vi "Windows Main-forextreme.vi"() -> ()   [LabVIEW 2016]
uses:
  <resource>/objmgr/ni.dex.rc
panel:
  out "Array 10":i32[][](array[numeric])
  in  "停止应用程序 11":bool
  in  "停止应用程序 10":bool
  out "Array 9":i32[][](array[numeric])
  in  "停止应用程序 9":bool
  out "Gaussian2-4":T1(plugin-control)
  out "Array 8":i32[][](array[numeric])
  in  "停止应用程序 8":bool
  out "Gaussian2-3":T1(plugin-control)
  out "Array 7":i32[][](array[numeric])
  in  "停止应用程序 7":bool
  out "Gaussian2-2":T1(plugin-control)
  out "Array 6":i32[][](array[numeric])
  in  "停止应用程序 6":bool
  out "Gaussian2-1":T1(plugin-control)
  out "Array 5":i32[][](array[numeric])
  in  "停止应用程序 5":bool
  out "Gaussian1-4":T1(plugin-control)
  out "Array 4":i32[][](array[numeric])
  in  "停止应用程序 4":bool
  out "Gaussian1-3":T1(plugin-control)
  out "Array 3":i32[][](array[numeric])
  in  "停止应用程序 3":bool
  out "Gaussian1-2":T1(plugin-control)
  out "Array 2":i32[][](array[numeric])
  out "error out 2":errorcluster
  in  "停止应用程序 2":bool
  out "OriImage":T1(plugin-control)
  out "Array":i32[][](array[numeric])
  out "Numeric":i32
  in  "终端IP地址":string
  out "error out":errorcluster
  in  "停止应用程序":bool
  out "Gaussian1-1":T1(plugin-control)
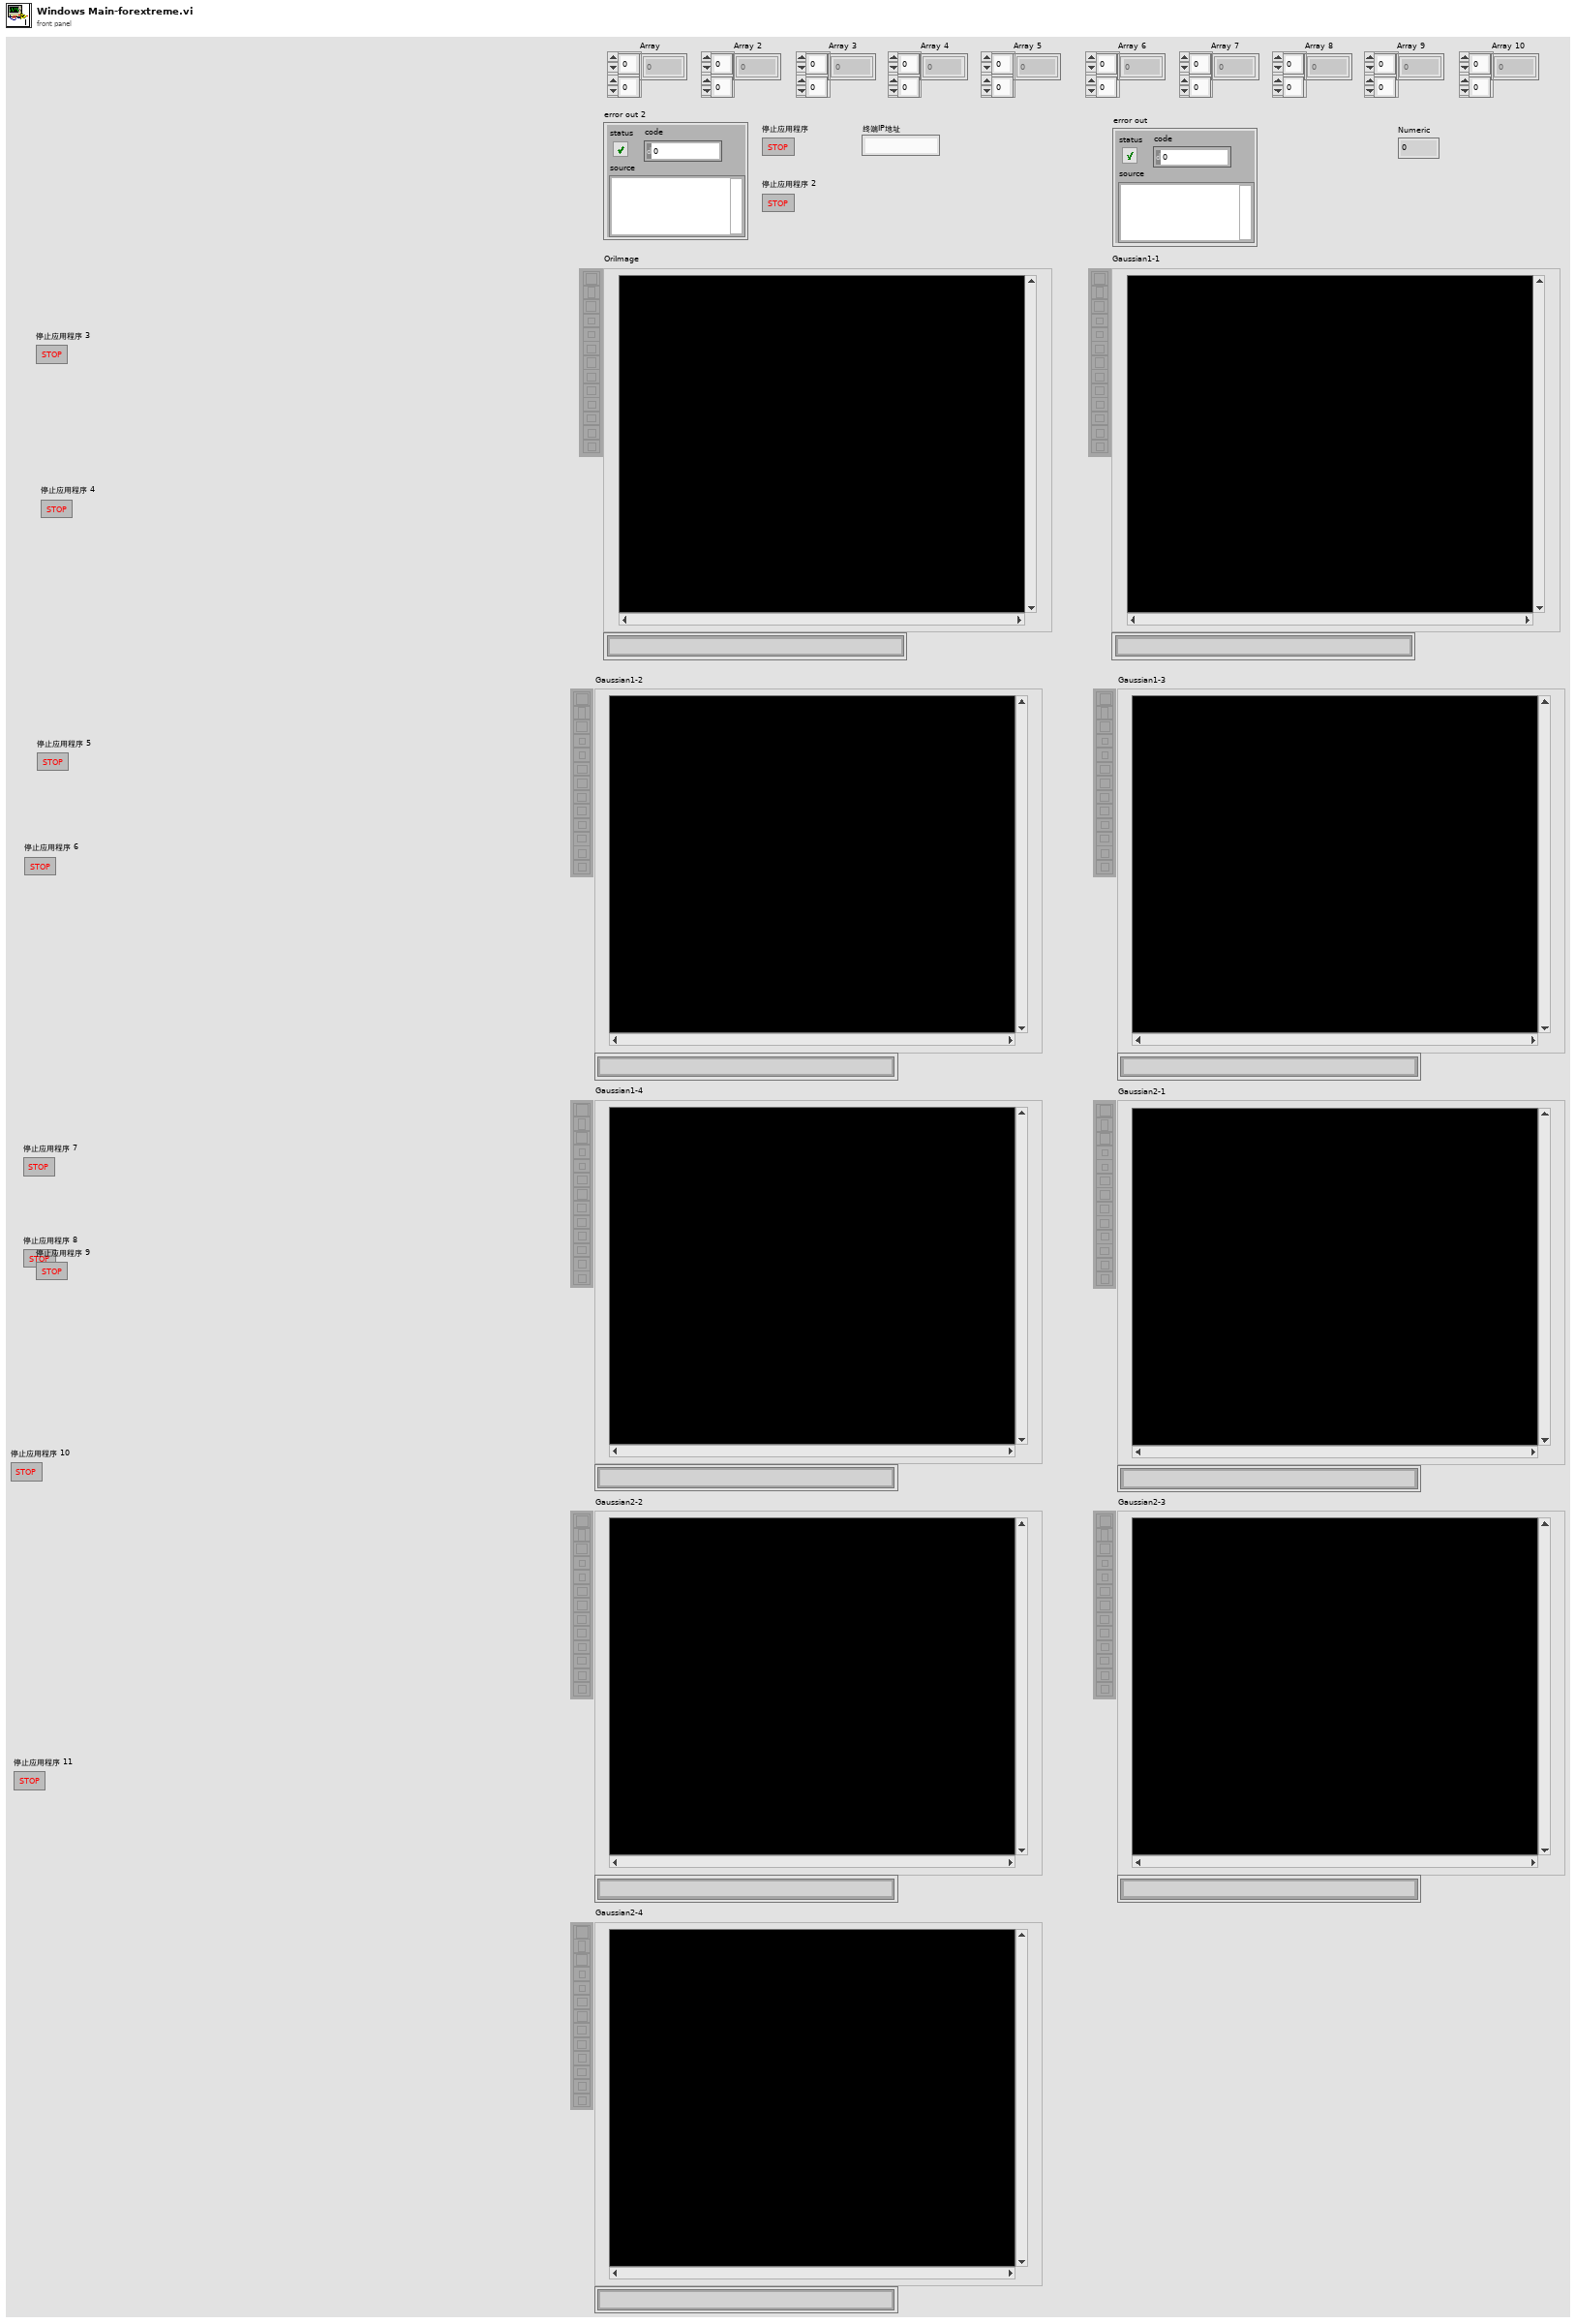
[diagram p1: front panel]
types:
  T1 = typedef "IMAQ Image.ctl" = refnum<image>
  T2 = typedef "Image Type" = u32
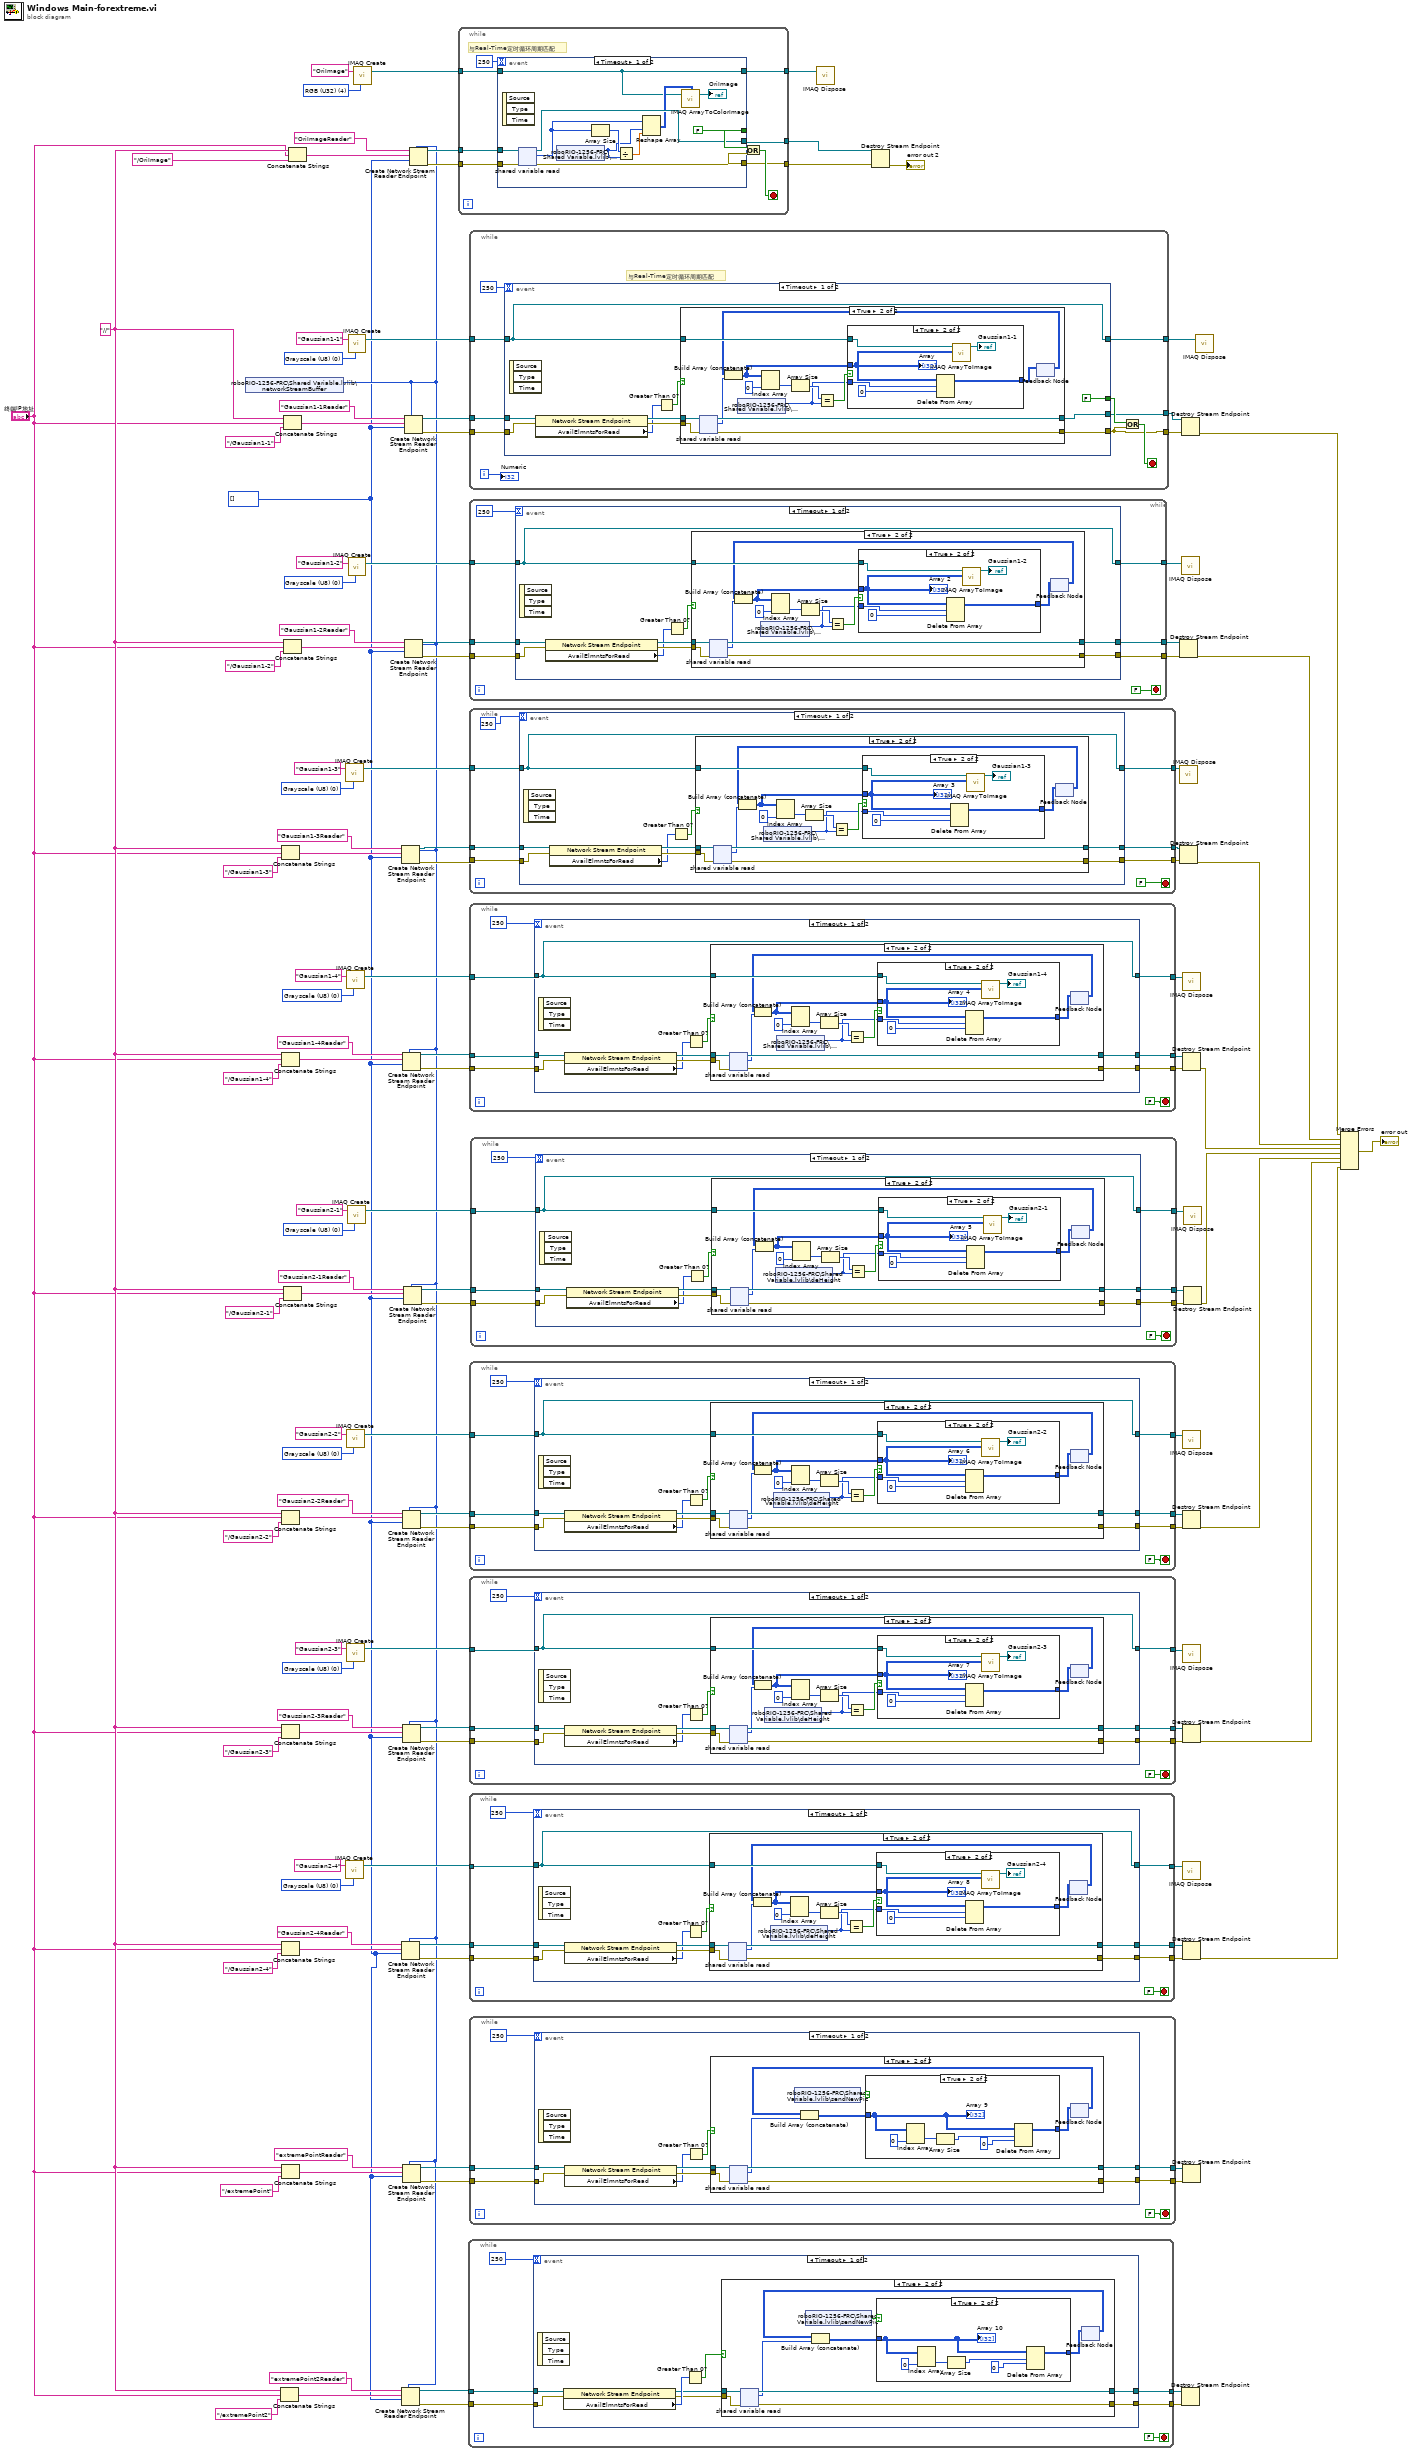
[diagram p0: block diagram]
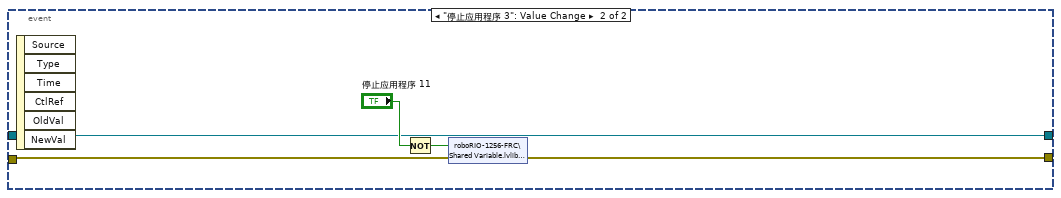
[diagram p4: hidden frame]
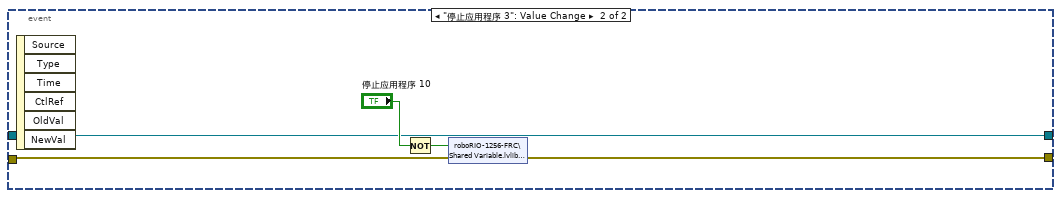
[diagram p7: hidden frame]
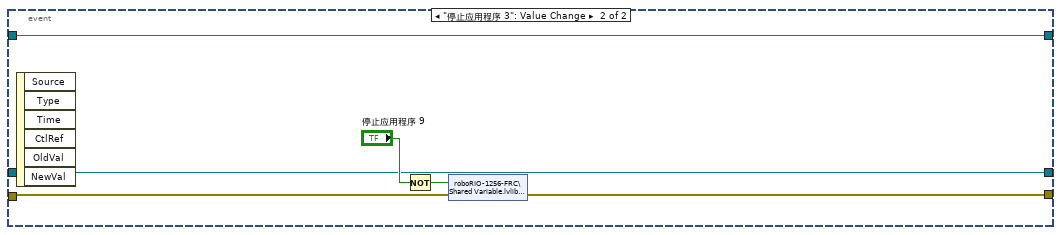
[diagram p10: hidden frame]
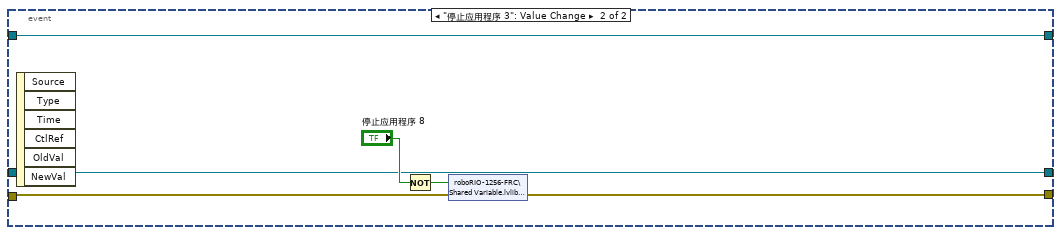
[diagram p13: hidden frame]
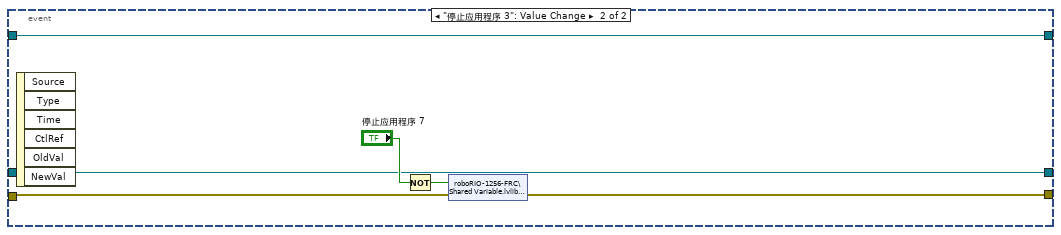
[diagram p16: hidden frame]
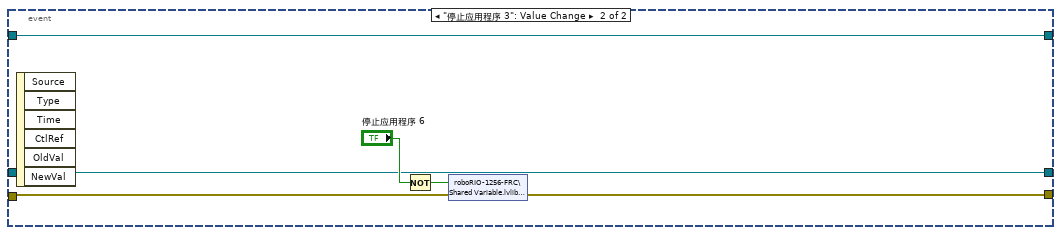
[diagram p19: hidden frame]
diagram:
  w32 = T2 0 items=["Grayscale (U8)", "Grayscale (I16)", "Grayscale (SGL)", "Complex (CSG)", "RGB (U32)", "HSL (U32)", "RGB (U64)", "Grayscale (U16)"] ("Image Type")
  w33 = T2 0 items=["Grayscale (U8)", "Grayscale (I16)", "Grayscale (SGL)", "Complex (CSG)", "RGB (U32)", "HSL (U32)", "RGB (U64)", "Grayscale (U16)"] ("Image Type")
  w54 = T2 0 items=["Grayscale (U8)", "Grayscale (I16)", "Grayscale (SGL)", "Complex (CSG)", "RGB (U32)", "HSL (U32)", "RGB (U64)", "Grayscale (U16)"] ("Image Type")
  w56 = T2 0 items=["Grayscale (U8)", "Grayscale (I16)", "Grayscale (SGL)", "Complex (CSG)", "RGB (U32)", "HSL (U32)", "RGB (U64)", "Grayscale (U16)"] ("Image Type")
  w90 = T2 0 items=["Grayscale (U8)", "Grayscale (I16)", "Grayscale (SGL)", "Complex (CSG)", "RGB (U32)", "HSL (U32)", "RGB (U64)", "Grayscale (U16)"] ("Image Type")
  w95 = T2 0 items=["Grayscale (U8)", "Grayscale (I16)", "Grayscale (SGL)", "Complex (CSG)", "RGB (U32)", "HSL (U32)", "RGB (U64)", "Grayscale (U16)"] ("Image Type")
  w96 = T2 0 items=["Grayscale (U8)", "Grayscale (I16)", "Grayscale (SGL)", "Complex (CSG)", "RGB (U32)", "HSL (U32)", "RGB (U64)", "Grayscale (U16)"] ("Image Type")
  w108 = T2 4 items=["Grayscale (U8)", "Grayscale (I16)", "Grayscale (SGL)", "Complex (CSG)", "RGB (U32)", "HSL (U32)", "RGB (U64)", "Grayscale (U16)"] ("Image Type")
  w101 = T2 0 items=["Grayscale (U8)", "Grayscale (I16)", "Grayscale (SGL)", "Complex (CSG)", "RGB (U32)", "HSL (U32)", "RGB (U64)", "Grayscale (U16)"] ("Image Type")
  w3 = i32[] []
  w2 = "//" ("string")
  n1 = shared-variable "roboRIO-1256-FRC\\Shared Variable.lvlib\\networkStreamBuffer"() -> (w4:i8)  [unwired: 1 in, 1 out]
  n2 = Concatenate Strings(w2, "终端IP地址", "/extremePoint2" ("string")) -> (w9:string)
  n3 = Concatenate Strings(w2, "终端IP地址", "/Gaussian1-3" ("string")) -> (w99:string)
  n4 = Concatenate Strings(w2, "终端IP地址", "/Gaussian2-4" ("string")) -> (w29:string)
  n5 = Concatenate Strings(w2, "终端IP地址", "/Gaussian1-4" ("string")) -> (w87:string)
  n6 = Concatenate Strings(w2, "终端IP地址", "/Gaussian2-2" ("string")) -> (w51:string)
  n7 = Concatenate Strings(w2, "终端IP地址", "/Gaussian2-3" ("string")) -> (w36:string)
  n8 = Concatenate Strings(w2, "终端IP地址", "/extremePoint" ("string")) -> (w14:string)
  n9 = Concatenate Strings(w2, "终端IP地址", "/Gaussian2-1" ("string")) -> (w59:string)
  n10 = Concatenate Strings(w2, "终端IP地址", "/Gaussian1-1" ("string")) -> (w124:string)
  n11 = Concatenate Strings(w2, "终端IP地址", "/Gaussian1-2" ("string")) -> (w103:string)
  n12 = Concatenate Strings(w2, "终端IP地址", "/OriImage" ("string")) -> (w114:string)
  n13 = call "IMAQ Create"("Image Name"="Gaussian1-3", "Image Type"=w95) -> ("New Image"=w78:T1)  [unwired: 3 in, 1 out]
  n14 = call "IMAQ Create"("Image Name"="Gaussian2-4", "Image Type"=w32) -> ("New Image"=w27:T1)  [unwired: 3 in, 1 out]
  n15 = call "IMAQ Create"("Image Name"="Gaussian1-4", "Image Type"=w90) -> ("New Image"=w84:T1)  [unwired: 3 in, 1 out]
  n16 = call "IMAQ Create"("Image Name"="Gaussian2-2", "Image Type"=w54) -> ("New Image"=w49:T1)  [unwired: 3 in, 1 out]
  n17 = call "IMAQ Create"("Image Name"="Gaussian2-3", "Image Type"=w33) -> ("New Image"=w38:T1)  [unwired: 3 in, 1 out]
  n18 = call "IMAQ Create"("Image Name"="Gaussian2-1", "Image Type"=w56) -> ("New Image"=w61:T1)  [unwired: 3 in, 1 out]
  n19 = call "IMAQ Create"("Image Name"="Gaussian1-1", "Image Type"=w101) -> ("New Image"=w120:T1)  [unwired: 3 in, 1 out]
  n20 = call "IMAQ Create"("Image Name"="Gaussian1-2", "Image Type"=w96) -> ("New Image"=w70:T1)  [unwired: 3 in, 1 out]
  n21 = call "IMAQ Create"("Image Name"="OriImage", "Image Type"=w108) -> ("New Image"=w107:T1)  [unwired: 3 in, 1 out]
  n22 = Create Network Stream Reader Endpoint(7:w4, 9:w3, 10:w9, 11:"extremePoint2Reader" ("reader name")) -> (0:w7:errorcluster, 3:w8:refnum<k21>)  [unwired: 3 in]
  n23 = Create Network Stream Reader Endpoint(7:w4, 9:w3, 10:w99, 11:"Gaussian1-3Reader" ("reader name")) -> (0:w76:errorcluster, 3:w77:refnum<k21>)  [unwired: 3 in]
  n24 = Create Network Stream Reader Endpoint(7:w4, 9:w3, 10:w29, 11:"Gaussian2-4Reader" ("reader name")) -> (0:w25:errorcluster, 3:w26:refnum<k21>)  [unwired: 3 in]
  n25 = Create Network Stream Reader Endpoint(7:w4, 9:w3, 10:w87, 11:"Gaussian1-4Reader" ("reader name")) -> (0:w82:errorcluster, 3:w83:refnum<k21>)  [unwired: 3 in]
  n26 = Create Network Stream Reader Endpoint(7:w4, 9:w3, 10:w51, 11:"Gaussian2-2Reader" ("reader name")) -> (0:w47:errorcluster, 3:w48:refnum<k21>)  [unwired: 3 in]
  n27 = Create Network Stream Reader Endpoint(7:w4, 9:w3, 10:w36, 11:"Gaussian2-3Reader" ("reader name")) -> (0:w40:errorcluster, 3:w39:refnum<k21>)  [unwired: 3 in]
  n28 = Create Network Stream Reader Endpoint(7:w4, 9:w3, 10:w14, 11:"extremePointReader" ("reader name")) -> (0:w16:errorcluster, 3:w15:refnum<k21>)  [unwired: 3 in]
  n29 = Create Network Stream Reader Endpoint(7:w4, 9:w3, 10:w59, 11:"Gaussian2-1Reader" ("reader name")) -> (0:w63:errorcluster, 3:w62:refnum<k21>)  [unwired: 3 in]
  n30 = Create Network Stream Reader Endpoint(7:w4, 9:w3, 10:w124, 11:"Gaussian1-1Reader" ("reader name")) -> (0:w127:errorcluster, 3:w118:refnum<k21>)  [unwired: 3 in]
  n31 = Create Network Stream Reader Endpoint(7:w4, 9:w3, 10:w103, 11:"Gaussian1-2Reader" ("reader name")) -> (0:w71:errorcluster, 3:w72:refnum<k21>)  [unwired: 3 in]
  n32 = Create Network Stream Reader Endpoint(7:w4, 9:w3, 10:w114, 11:"OriImageReader" ("reader name")) -> (0:w117:errorcluster, 3:w112:refnum<k21>)  [unwired: 3 in]
  n33 = while {
    tunnel: w112 -> [w131]
    tunnel: [w130] -> w111
    tunnel: w107 -> [w129]
    tunnel: [w128] -> w106
    tunnel: w117 -> [w133]
    tunnel: [w132] -> w113
    stop <- w134 stop-if-true
    # "与Real-Time定时循环周期匹配"
    n34 = event shown="[0] Timeout" {
      selector: _ -> [_ _]
      dyn-events: _ -> [_ _]
      timeout: 250 -> [_ _]
      tunnel: [FALSE ("停止应用程序") "停止应用程序 2"] -> w135
      tunnel: w133 -> [w148 w152]
      tunnel: [w147 w151] -> w132
      tunnel: w131 -> [w146 w149]
      tunnel: [w145 w149] -> w130
      tunnel: w129 -> [w138 w150]
      tunnel: [w138 w150] -> w128
      event Timeout {
        n35 = event-data() -> ()  [unwired: 1 in, 3 out]
        n36 = shared-variable-read(w146, w148) -> (w145:refnum<k21>, w147:errorcluster, w141:i32[])  [unwired: 1 in, 1 out]
        n37 = shared-variable "roboRIO-1256-FRC\\Shared Variable.lvlib\\Height"() -> (w137:u16)  [unwired: 1 in, 1 out]
        n38 = Array Size(array=w141) -> (size(s)=w143:i32)
        n39 = Divide(x=w143, y=w137) -> (x/y=w142:dbl)
        n40 = Reshape Array(w141, w137, w142) -> (w140:i32[][])
        n41 = call "IMAQ ArrayToColorImage"("Image Pixels (U32)"=w140, "Image"=w138) -> ("Image Out"=→"OriImage":T1)  [unwired: 3 in, 1 out]
      }
      event "停止应用程序 2": Value Change {
        n42 = event-data() -> ()  [unwired: 1 in, 6 out]
        n43 = Not(x="停止应用程序 2") -> (.not. x?=w153:bool)
        n44 = shared-variable "roboRIO-1256-FRC\\Shared Variable.lvlib\\Active"(w153, error in=w152) -> (error out=w151:errorcluster)
      }
    }
    n45 = Or(x=w135, y=w132) -> (x .or. y?=w134:bool)
  }
  n46 = while {
    tunnel: w8 -> [w160]
    tunnel: [w157] -> w5
    tunnel: w7 -> [w159]
    tunnel: [w158] -> w6
    stop <- FALSE stop-if-true
    n47 = event shown="[0] Timeout" {
      selector: _ -> [_ _]
      dyn-events: _ -> [_ _]
      timeout: 250 -> [_ _]
      tunnel: w159 -> [w168 w189]
      tunnel: [w161 w188] -> w158
      tunnel: w160 -> [w167 w187]
      tunnel: [w162 w187] -> w157
      event Timeout {
        n48 = event-data() -> ()  [unwired: 1 in, 3 out]
        n49 = property class="Network Stream Endpoint"(reference=w167, error in=w168) -> (reference out=w165:refnum<k21>, error out=w164:errorcluster, "AvailElmntsForRead"=w166:i32)
        n50 = Greater Than 0?(x=w166) -> (x > 0?=w163:bool)
        n51 = case shown="True" w163 {
          tunnel: [w169 w179] -> w161
          tunnel: [w170 w178] -> w162
          tunnel: w164 -> [w169 w177]
          tunnel: w165 -> [w170 w176]
          frame False {
          }
          frame True {
            n52 = shared-variable-read(w176, w177) -> (w178:refnum<k21>, w179:errorcluster, w175:i32[])  [unwired: 1 in, 1 out]
            n53 = shared-variable "roboRIO-1256-FRC\\Shared Variable.lvlib\\sendNewPic"() -> (w171:bool)  [unwired: 1 in, 1 out]
            n54 = feedback #1() -> (w173:i32[][])  [unwired: 1 in]
            n55 = Build Array (concatenate)(w173, w175) -> (w172:i32[][])
            n56 = case shown="True" w171 {
              tunnel: w172 -> [w180 w181]
              tunnel: [w180 w185] -> w174
              frame False {
              }
              frame True {
                n57 = Index Array(array=w181, index (col)=0 ("disabled index (col)")) -> (element=w184:i32[])  [unwired: 1 in]
                n58 = Array Size(array=w184) -> (size(s)=w182:i32)
                n59 = Delete From Array(array=w181, length=w182, index (row)=0) -> (array with subset deleted=w185:i32[][])  [unwired: 1 in, 1 out]
                "Array 10" <- w181
              }
            }
            n60 = feedback-in #1(w174) -> ()
          }
        }
      }
      event "停止应用程序 3": Value Change {
        n61 = event-data() -> ()  [unwired: 1 in, 6 out]
        n62 = Not(x="停止应用程序 11") -> (.not. x?=w190:bool)
        n63 = shared-variable "roboRIO-1256-FRC\\Shared Variable.lvlib\\Active"(w190, error in=w189) -> (error out=w188:errorcluster)
      }
    }
  }
  n64 = while {
    tunnel: w27 -> [w199]
    tunnel: [w194] -> w22
    tunnel: w26 -> [w198]
    tunnel: [w195] -> w23
    tunnel: w25 -> [w197]
    tunnel: [w196] -> w24
    stop <- FALSE stop-if-true
    n65 = event shown="[0] Timeout" {
      selector: _ -> [_ _]
      dyn-events: _ -> [_ _]
      timeout: 250 -> [_ _]
      tunnel: w197 -> [w205 w235]
      tunnel: [w208 w234] -> w196
      tunnel: w198 -> [w204 w232]
      tunnel: [w207 w232] -> w195
      tunnel: w199 -> [w206 w233]
      tunnel: [w206 w233] -> w194
      event Timeout {
        n66 = event-data() -> ()  [unwired: 1 in, 3 out]
        n67 = property class="Network Stream Endpoint"(reference=w204, error in=w205) -> (reference out=w202:refnum<k21>, error out=w203:errorcluster, "AvailElmntsForRead"=w201:i32)
        n68 = Greater Than 0?(x=w201) -> (x > 0?=w200:bool)
        n69 = case shown="True" w200 {
          tunnel: [w209 w224] -> w208
          tunnel: [w210 w223] -> w207
          tunnel: w206 -> [_ w216]
          tunnel: w203 -> [w209 w218]
          tunnel: w202 -> [w210 w217]
          frame False {
          }
          frame True {
            n70 = shared-variable-read(w217, w218) -> (w223:refnum<k21>, w224:errorcluster, w214:i32[])  [unwired: 1 in, 1 out]
            n71 = shared-variable "roboRIO-1256-FRC\\Shared Variable.lvlib\\deHeight"() -> (w211:u16)  [unwired: 1 in, 1 out]
            n72 = feedback #2() -> (w212:i32[][])  [unwired: 1 in]
            n73 = Build Array (concatenate)(w212, w214) -> (w215:i32[][])
            n74 = Index Array(array=w215, index (col)=0 ("disabled index (col)")) -> (element=w221:i32[])  [unwired: 1 in]
            n75 = Array Size(array=w221) -> (size(s)=w220:i32)
            n76 = Equal?(x=w220, y=w211) -> (x = y?=w219:bool)
            n77 = case shown="True" w219 {
              tunnel: w215 -> [w225 w226]
              tunnel: [w225 w227] -> w213
              tunnel: w211 -> [_ w231]
              tunnel: w216 -> [_ w228]
              frame False {
              }
              frame True {
                n78 = Delete From Array(array=w226, length=w231, index (row)=0) -> (array with subset deleted=w227:i32[][])  [unwired: 1 in, 1 out]
                n79 = call "IMAQ ArrayToImage"("Image Pixels (U8)"=w226, "Image"=w228) -> ("Image Out"=→"Gaussian2-4":T1)  [unwired: 8 in, 1 out]
                "Array 8" <- w226
              }
            }
            n80 = feedback-in #2(w213) -> ()
          }
        }
      }
      event "停止应用程序 3": Value Change {
        n81 = event-data() -> ()  [unwired: 1 in, 6 out]
        n82 = Not(x="停止应用程序 9") -> (.not. x?=w236:bool)
        n83 = shared-variable "roboRIO-1256-FRC\\Shared Variable.lvlib\\Active"(w236, error in=w235) -> (error out=w234:errorcluster)
      }
    }
  }
  n84 = while {
    tunnel: w118 -> [w242]
    tunnel: [w241] -> w122
    tunnel: w120 -> [w240]
    tunnel: [w239] -> w119
    tunnel: w127 -> [w244]
    tunnel: [w243] -> w123
    i -> [w238]
    stop <- w245 stop-if-true
    # "与Real-Time定时循环周期匹配"
    n85 = event shown="[0] Timeout" {
      selector: _ -> [_ _]
      dyn-events: _ -> [_ _]
      timeout: 250 -> [_ _]
      tunnel: [FALSE ("停止应用程序") "停止应用程序"] -> w246
      tunnel: w244 -> [w253 w284]
      tunnel: [w257 w283] -> w243
      tunnel: w242 -> [w252 w281]
      tunnel: [w256 w281] -> w241
      tunnel: w240 -> [w254 w282]
      tunnel: [w254 w282] -> w239
      event Timeout {
        n86 = event-data() -> ()  [unwired: 1 in, 3 out]
        n87 = property class="Network Stream Endpoint"(reference=w252, error in=w253) -> (reference out=w250:refnum<k21>, error out=w251:errorcluster, "AvailElmntsForRead"=w249:i32)
        n88 = Greater Than 0?(x=w249) -> (x > 0?=w248:bool)
        n89 = case shown="True" w248 {
          tunnel: [w258 w273] -> w257
          tunnel: [w259 w272] -> w256
          tunnel: w254 -> [_ w265]
          tunnel: w251 -> [w258 w267]
          tunnel: w250 -> [w259 w266]
          frame False {
          }
          frame True {
            n90 = shared-variable-read(w266, w267) -> (w272:refnum<k21>, w273:errorcluster, w263:i32[])  [unwired: 1 in, 1 out]
            n91 = shared-variable "roboRIO-1256-FRC\\Shared Variable.lvlib\\Height"() -> (w260:u16)  [unwired: 1 in, 1 out]
            n92 = feedback #3() -> (w261:i32[][])  [unwired: 1 in]
            n93 = Build Array (concatenate)(w261, w263) -> (w264:i32[][])
            n94 = Index Array(array=w264, index (col)=0 ("disabled index (col)")) -> (element=w270:i32[])  [unwired: 1 in]
            n95 = Array Size(array=w270) -> (size(s)=w269:i32)
            n96 = Equal?(x=w269, y=w260) -> (x = y?=w268:bool)
            n97 = case shown="True" w268 {
              tunnel: w264 -> [w274 w275]
              tunnel: [w274 w276] -> w262
              tunnel: w260 -> [_ w280]
              tunnel: w265 -> [_ w277]
              frame False {
              }
              frame True {
                n98 = Delete From Array(array=w275, length=w280, index (row)=0) -> (array with subset deleted=w276:i32[][])  [unwired: 1 in, 1 out]
                n99 = call "IMAQ ArrayToImage"("Image Pixels (U8)"=w275, "Image"=w277) -> ("Image Out"=→"Gaussian1-1":T1)  [unwired: 8 in, 1 out]
                "Array" <- w275
              }
            }
            n100 = feedback-in #3(w262) -> ()
          }
        }
      }
      event "停止应用程序": Value Change {
        n101 = event-data() -> ()  [unwired: 1 in, 6 out]
        n102 = Not(x="停止应用程序") -> (.not. x?=w285:bool)
        n103 = shared-variable "roboRIO-1256-FRC\\Shared Variable.lvlib\\Active"(w285, error in=w284) -> (error out=w283:errorcluster)
      }
    }
    n104 = Or(x=w246, y=w243) -> (x .or. y?=w245:bool)
    "Numeric" <- w238
  }
  n105 = while {
    tunnel: w70 -> [w292]
    tunnel: [w291] -> w69
    tunnel: w72 -> [w294]
    tunnel: [w290] -> w68
    tunnel: w71 -> [w293]
    tunnel: [w289] -> w67
    stop <- FALSE stop-if-true
    n106 = event shown="[0] Timeout" {
      selector: _ -> [_ _]
      dyn-events: _ -> [_ _]
      timeout: 250 -> [_ _]
      tunnel: w293 -> [w300 w330]
      tunnel: [w303 w329] -> w289
      tunnel: w294 -> [w299 w327]
      tunnel: [w302 w327] -> w290
      tunnel: w292 -> [w301 w328]
      tunnel: [w301 w328] -> w291
      event Timeout {
        n107 = event-data() -> ()  [unwired: 1 in, 3 out]
        n108 = property class="Network Stream Endpoint"(reference=w299, error in=w300) -> (reference out=w297:refnum<k21>, error out=w298:errorcluster, "AvailElmntsForRead"=w296:i32)
        n109 = Greater Than 0?(x=w296) -> (x > 0?=w295:bool)
        n110 = case shown="True" w295 {
          tunnel: [w304 w319] -> w303
          tunnel: [w305 w318] -> w302
          tunnel: w301 -> [_ w311]
          tunnel: w298 -> [w304 w313]
          tunnel: w297 -> [w305 w312]
          frame False {
          }
          frame True {
            n111 = shared-variable-read(w312, w313) -> (w318:refnum<k21>, w319:errorcluster, w309:i32[])  [unwired: 1 in, 1 out]
            n112 = shared-variable "roboRIO-1256-FRC\\Shared Variable.lvlib\\Height"() -> (w306:u16)  [unwired: 1 in, 1 out]
            n113 = feedback #4() -> (w307:i32[][])  [unwired: 1 in]
            n114 = Build Array (concatenate)(w307, w309) -> (w310:i32[][])
            n115 = Index Array(array=w310, index (col)=0 ("disabled index (col)")) -> (element=w316:i32[])  [unwired: 1 in]
            n116 = Array Size(array=w316) -> (size(s)=w315:i32)
            n117 = Equal?(x=w315, y=w306) -> (x = y?=w314:bool)
            n118 = case shown="True" w314 {
              tunnel: w310 -> [w320 w321]
              tunnel: [w320 w322] -> w308
              tunnel: w306 -> [_ w326]
              tunnel: w311 -> [_ w323]
              frame False {
              }
              frame True {
                n119 = Delete From Array(array=w321, length=w326, index (row)=0) -> (array with subset deleted=w322:i32[][])  [unwired: 1 in, 1 out]
                n120 = call "IMAQ ArrayToImage"("Image Pixels (U8)"=w321, "Image"=w323) -> ("Image Out"=→"Gaussian1-2":T1)  [unwired: 8 in, 1 out]
                "Array 2" <- w321
              }
            }
            n121 = feedback-in #4(w308) -> ()
          }
        }
      }
      event "停止应用程序 3": Value Change {
        n122 = event-data() -> ()  [unwired: 1 in, 6 out]
        n123 = Not(x="停止应用程序 3") -> (.not. x?=w331:bool)
        n124 = shared-variable "roboRIO-1256-FRC\\Shared Variable.lvlib\\Active"(w331, error in=w330) -> (error out=w329:errorcluster)
      }
    }
  }
  n125 = while {
    tunnel: w78 -> [w340]
    tunnel: [w335] -> w73
    tunnel: w77 -> [w339]
    tunnel: [w337] -> w75
    tunnel: w76 -> [w338]
    tunnel: [w336] -> w74
    stop <- FALSE stop-if-true
    n126 = event shown="[0] Timeout" {
      selector: _ -> [_ _]
      dyn-events: _ -> [_ _]
      timeout: 250 -> [_ _]
      tunnel: w338 -> [w346 w376]
      tunnel: [w349 w375] -> w336
      tunnel: w339 -> [w345 w373]
      tunnel: [w348 w373] -> w337
      tunnel: w340 -> [w347 w374]
      tunnel: [w347 w374] -> w335
      event Timeout {
        n127 = event-data() -> ()  [unwired: 1 in, 3 out]
        n128 = property class="Network Stream Endpoint"(reference=w345, error in=w346) -> (reference out=w343:refnum<k21>, error out=w344:errorcluster, "AvailElmntsForRead"=w342:i32)
        n129 = Greater Than 0?(x=w342) -> (x > 0?=w341:bool)
        n130 = case shown="True" w341 {
          tunnel: [w350 w365] -> w349
          tunnel: [w351 w364] -> w348
          tunnel: w347 -> [_ w357]
          tunnel: w344 -> [w350 w359]
          tunnel: w343 -> [w351 w358]
          frame False {
          }
          frame True {
            n131 = shared-variable-read(w358, w359) -> (w364:refnum<k21>, w365:errorcluster, w355:i32[])  [unwired: 1 in, 1 out]
            n132 = shared-variable "roboRIO-1256-FRC\\Shared Variable.lvlib\\Height"() -> (w352:u16)  [unwired: 1 in, 1 out]
            n133 = feedback #5() -> (w353:i32[][])  [unwired: 1 in]
            n134 = Build Array (concatenate)(w353, w355) -> (w356:i32[][])
            n135 = Index Array(array=w356, index (col)=0 ("disabled index (col)")) -> (element=w362:i32[])  [unwired: 1 in]
            n136 = Array Size(array=w362) -> (size(s)=w361:i32)
            n137 = Equal?(x=w361, y=w352) -> (x = y?=w360:bool)
            n138 = case shown="True" w360 {
              tunnel: w356 -> [w366 w367]
              tunnel: [w366 w368] -> w354
              tunnel: w352 -> [_ w372]
              tunnel: w357 -> [_ w369]
              frame False {
              }
              frame True {
                n139 = Delete From Array(array=w367, length=w372, index (row)=0) -> (array with subset deleted=w368:i32[][])  [unwired: 1 in, 1 out]
                n140 = call "IMAQ ArrayToImage"("Image Pixels (U8)"=w367, "Image"=w369) -> ("Image Out"=→"Gaussian1-3":T1)  [unwired: 8 in, 1 out]
                "Array 3" <- w367
              }
            }
            n141 = feedback-in #5(w354) -> ()
          }
        }
      }
      event "停止应用程序 3": Value Change {
        n142 = event-data() -> ()  [unwired: 1 in, 6 out]
        n143 = Not(x="停止应用程序 4") -> (.not. x?=w377:bool)
        n144 = shared-variable "roboRIO-1256-FRC\\Shared Variable.lvlib\\Active"(w377, error in=w376) -> (error out=w375:errorcluster)
      }
    }
  }
  n145 = while {
    tunnel: w84 -> [w386]
    tunnel: [w381] -> w79
    tunnel: w83 -> [w385]
    tunnel: [w382] -> w80
    tunnel: w82 -> [w384]
    tunnel: [w383] -> w81
    stop <- FALSE stop-if-true
    n146 = event shown="[0] Timeout" {
      selector: _ -> [_ _]
      dyn-events: _ -> [_ _]
      timeout: 250 -> [_ _]
      tunnel: w384 -> [w392 w422]
      tunnel: [w395 w421] -> w383
      tunnel: w385 -> [w391 w419]
      tunnel: [w394 w419] -> w382
      tunnel: w386 -> [w393 w420]
      tunnel: [w393 w420] -> w381
      event Timeout {
        n147 = event-data() -> ()  [unwired: 1 in, 3 out]
        n148 = property class="Network Stream Endpoint"(reference=w391, error in=w392) -> (reference out=w389:refnum<k21>, error out=w390:errorcluster, "AvailElmntsForRead"=w388:i32)
        n149 = Greater Than 0?(x=w388) -> (x > 0?=w387:bool)
        n150 = case shown="True" w387 {
          tunnel: [w396 w411] -> w395
          tunnel: [w397 w410] -> w394
          tunnel: w393 -> [_ w403]
          tunnel: w390 -> [w396 w405]
          tunnel: w389 -> [w397 w404]
          frame False {
          }
          frame True {
            n151 = shared-variable-read(w404, w405) -> (w410:refnum<k21>, w411:errorcluster, w401:i32[])  [unwired: 1 in, 1 out]
            n152 = shared-variable "roboRIO-1256-FRC\\Shared Variable.lvlib\\Height"() -> (w398:u16)  [unwired: 1 in, 1 out]
            n153 = feedback #6() -> (w399:i32[][])  [unwired: 1 in]
            n154 = Build Array (concatenate)(w399, w401) -> (w402:i32[][])
            n155 = Index Array(array=w402, index (col)=0 ("disabled index (col)")) -> (element=w408:i32[])  [unwired: 1 in]
            n156 = Array Size(array=w408) -> (size(s)=w407:i32)
            n157 = Equal?(x=w407, y=w398) -> (x = y?=w406:bool)
            n158 = case shown="True" w406 {
              tunnel: w402 -> [w412 w413]
              tunnel: [w412 w414] -> w400
              tunnel: w398 -> [_ w418]
              tunnel: w403 -> [_ w415]
              frame False {
              }
              frame True {
                n159 = Delete From Array(array=w413, length=w418, index (row)=0) -> (array with subset deleted=w414:i32[][])  [unwired: 1 in, 1 out]
                n160 = call "IMAQ ArrayToImage"("Image Pixels (U8)"=w413, "Image"=w415) -> ("Image Out"=→"Gaussian1-4":T1)  [unwired: 8 in, 1 out]
                "Array 4" <- w413
              }
            }
            n161 = feedback-in #6(w400) -> ()
          }
        }
      }
      event "停止应用程序 3": Value Change {
        n162 = event-data() -> ()  [unwired: 1 in, 6 out]
        n163 = Not(x="停止应用程序 5") -> (.not. x?=w423:bool)
        n164 = shared-variable "roboRIO-1256-FRC\\Shared Variable.lvlib\\Active"(w423, error in=w422) -> (error out=w421:errorcluster)
      }
    }
  }
  n165 = while {
    tunnel: w49 -> [w432]
    tunnel: [w427] -> w44
    tunnel: w48 -> [w431]
    tunnel: [w428] -> w45
    tunnel: w47 -> [w430]
    tunnel: [w429] -> w46
    stop <- FALSE stop-if-true
    n166 = event shown="[0] Timeout" {
      selector: _ -> [_ _]
      dyn-events: _ -> [_ _]
      timeout: 250 -> [_ _]
      tunnel: w430 -> [w438 w468]
      tunnel: [w441 w467] -> w429
      tunnel: w431 -> [w437 w465]
      tunnel: [w440 w465] -> w428
      tunnel: w432 -> [w439 w466]
      tunnel: [w439 w466] -> w427
      event Timeout {
        n167 = event-data() -> ()  [unwired: 1 in, 3 out]
        n168 = property class="Network Stream Endpoint"(reference=w437, error in=w438) -> (reference out=w435:refnum<k21>, error out=w436:errorcluster, "AvailElmntsForRead"=w434:i32)
        n169 = Greater Than 0?(x=w434) -> (x > 0?=w433:bool)
        n170 = case shown="True" w433 {
          tunnel: [w442 w457] -> w441
          tunnel: [w443 w456] -> w440
          tunnel: w439 -> [_ w449]
          tunnel: w436 -> [w442 w451]
          tunnel: w435 -> [w443 w450]
          frame False {
          }
          frame True {
            n171 = shared-variable-read(w450, w451) -> (w456:refnum<k21>, w457:errorcluster, w447:i32[])  [unwired: 1 in, 1 out]
            n172 = shared-variable "roboRIO-1256-FRC\\Shared Variable.lvlib\\deHeight"() -> (w444:u16)  [unwired: 1 in, 1 out]
            n173 = feedback #7() -> (w445:i32[][])  [unwired: 1 in]
            n174 = Build Array (concatenate)(w445, w447) -> (w448:i32[][])
            n175 = Index Array(array=w448, index (col)=0 ("disabled index (col)")) -> (element=w454:i32[])  [unwired: 1 in]
            n176 = Array Size(array=w454) -> (size(s)=w453:i32)
            n177 = Equal?(x=w453, y=w444) -> (x = y?=w452:bool)
            n178 = case shown="True" w452 {
              tunnel: w448 -> [w458 w459]
              tunnel: [w458 w460] -> w446
              tunnel: w444 -> [_ w464]
              tunnel: w449 -> [_ w461]
              frame False {
              }
              frame True {
                n179 = Delete From Array(array=w459, length=w464, index (row)=0) -> (array with subset deleted=w460:i32[][])  [unwired: 1 in, 1 out]
                n180 = call "IMAQ ArrayToImage"("Image Pixels (U8)"=w459, "Image"=w461) -> ("Image Out"=→"Gaussian2-2":T1)  [unwired: 8 in, 1 out]
                "Array 6" <- w459
              }
            }
            n181 = feedback-in #7(w446) -> ()
          }
        }
      }
      event "停止应用程序 3": Value Change {
        n182 = event-data() -> ()  [unwired: 1 in, 6 out]
        n183 = Not(x="停止应用程序 7") -> (.not. x?=w469:bool)
        n184 = shared-variable "roboRIO-1256-FRC\\Shared Variable.lvlib\\Active"(w469, error in=w468) -> (error out=w467:errorcluster)
      }
    }
  }
  n185 = while {
    tunnel: w38 -> [w478]
    tunnel: [w473] -> w43
    tunnel: w39 -> [w477]
    tunnel: [w474] -> w42
    tunnel: w40 -> [w476]
    tunnel: [w475] -> w41
    stop <- FALSE stop-if-true
    n186 = event shown="[0] Timeout" {
      selector: _ -> [_ _]
      dyn-events: _ -> [_ _]
      timeout: 250 -> [_ _]
      tunnel: w476 -> [w484 w514]
      tunnel: [w487 w513] -> w475
      tunnel: w477 -> [w483 w511]
      tunnel: [w486 w511] -> w474
      tunnel: w478 -> [w485 w512]
      tunnel: [w485 w512] -> w473
      event Timeout {
        n187 = event-data() -> ()  [unwired: 1 in, 3 out]
        n188 = property class="Network Stream Endpoint"(reference=w483, error in=w484) -> (reference out=w481:refnum<k21>, error out=w482:errorcluster, "AvailElmntsForRead"=w480:i32)
        n189 = Greater Than 0?(x=w480) -> (x > 0?=w479:bool)
        n190 = case shown="True" w479 {
          tunnel: [w488 w503] -> w487
          tunnel: [w489 w502] -> w486
          tunnel: w485 -> [_ w495]
          tunnel: w482 -> [w488 w497]
          tunnel: w481 -> [w489 w496]
          frame False {
          }
          frame True {
            n191 = shared-variable-read(w496, w497) -> (w502:refnum<k21>, w503:errorcluster, w493:i32[])  [unwired: 1 in, 1 out]
            n192 = shared-variable "roboRIO-1256-FRC\\Shared Variable.lvlib\\deHeight"() -> (w490:u16)  [unwired: 1 in, 1 out]
            n193 = feedback #8() -> (w491:i32[][])  [unwired: 1 in]
            n194 = Build Array (concatenate)(w491, w493) -> (w494:i32[][])
            n195 = Index Array(array=w494, index (col)=0 ("disabled index (col)")) -> (element=w500:i32[])  [unwired: 1 in]
            n196 = Array Size(array=w500) -> (size(s)=w499:i32)
            n197 = Equal?(x=w499, y=w490) -> (x = y?=w498:bool)
            n198 = case shown="True" w498 {
              tunnel: w494 -> [w504 w505]
              tunnel: [w504 w506] -> w492
              tunnel: w490 -> [_ w510]
              tunnel: w495 -> [_ w507]
              frame False {
              }
              frame True {
                n199 = Delete From Array(array=w505, length=w510, index (row)=0) -> (array with subset deleted=w506:i32[][])  [unwired: 1 in, 1 out]
                n200 = call "IMAQ ArrayToImage"("Image Pixels (U8)"=w505, "Image"=w507) -> ("Image Out"=→"Gaussian2-3":T1)  [unwired: 8 in, 1 out]
                "Array 7" <- w505
              }
            }
            n201 = feedback-in #8(w492) -> ()
          }
        }
      }
      event "停止应用程序 3": Value Change {
        n202 = event-data() -> ()  [unwired: 1 in, 6 out]
        n203 = Not(x="停止应用程序 8") -> (.not. x?=w515:bool)
        n204 = shared-variable "roboRIO-1256-FRC\\Shared Variable.lvlib\\Active"(w515, error in=w514) -> (error out=w513:errorcluster)
      }
    }
  }
  n205 = while {
    tunnel: w15 -> [w522]
    tunnel: [w519] -> w18
    tunnel: w16 -> [w521]
    tunnel: [w520] -> w17
    stop <- FALSE stop-if-true
    n206 = event shown="[0] Timeout" {
      selector: _ -> [_ _]
      dyn-events: _ -> [_ _]
      timeout: 250 -> [_ _]
      tunnel: w521 -> [w528 w551]
      tunnel: [w530 w550] -> w520
      tunnel: w522 -> [w527 w549]
      tunnel: [w529 w549] -> w519
      event Timeout {
        n207 = event-data() -> ()  [unwired: 1 in, 3 out]
        n208 = property class="Network Stream Endpoint"(reference=w527, error in=w528) -> (reference out=w525:refnum<k21>, error out=w526:errorcluster, "AvailElmntsForRead"=w524:i32)
        n209 = Greater Than 0?(x=w524) -> (x > 0?=w523:bool)
        n210 = case shown="True" w523 {
          tunnel: [w531 w541] -> w530
          tunnel: [w532 w540] -> w529
          tunnel: w526 -> [w531 w539]
          tunnel: w525 -> [w532 w538]
          frame False {
          }
          frame True {
            n211 = shared-variable-read(w538, w539) -> (w540:refnum<k21>, w541:errorcluster, w537:i32[])  [unwired: 1 in, 1 out]
            n212 = shared-variable "roboRIO-1256-FRC\\Shared Variable.lvlib\\sendNewPic"() -> (w533:bool)  [unwired: 1 in, 1 out]
            n213 = feedback #9() -> (w535:i32[][])  [unwired: 1 in]
            n214 = Build Array (concatenate)(w535, w537) -> (w534:i32[][])
            n215 = case shown="True" w533 {
              tunnel: w534 -> [w542 w543]
              tunnel: [w542 w547] -> w536
              frame False {
              }
              frame True {
                n216 = Index Array(array=w543, index (col)=0 ("disabled index (col)")) -> (element=w546:i32[])  [unwired: 1 in]
                n217 = Array Size(array=w546) -> (size(s)=w544:i32)
                n218 = Delete From Array(array=w543, length=w544, index (row)=0) -> (array with subset deleted=w547:i32[][])  [unwired: 1 in, 1 out]
                "Array 9" <- w543
              }
            }
            n219 = feedback-in #9(w536) -> ()
          }
        }
      }
      event "停止应用程序 3": Value Change {
        n220 = event-data() -> ()  [unwired: 1 in, 6 out]
        n221 = Not(x="停止应用程序 10") -> (.not. x?=w552:bool)
        n222 = shared-variable "roboRIO-1256-FRC\\Shared Variable.lvlib\\Active"(w552, error in=w551) -> (error out=w550:errorcluster)
      }
    }
  }
  n223 = while {
    tunnel: w61 -> [w561]
    tunnel: [w556] -> w66
    tunnel: w62 -> [w560]
    tunnel: [w557] -> w65
    tunnel: w63 -> [w559]
    tunnel: [w558] -> w64
    stop <- FALSE stop-if-true
    n224 = event shown="[0] Timeout" {
      selector: _ -> [_ _]
      dyn-events: _ -> [_ _]
      timeout: 250 -> [_ _]
      tunnel: w559 -> [w567 w597]
      tunnel: [w570 w596] -> w558
      tunnel: w560 -> [w566 w594]
      tunnel: [w569 w594] -> w557
      tunnel: w561 -> [w568 w595]
      tunnel: [w568 w595] -> w556
      event Timeout {
        n225 = event-data() -> ()  [unwired: 1 in, 3 out]
        n226 = property class="Network Stream Endpoint"(reference=w566, error in=w567) -> (reference out=w564:refnum<k21>, error out=w565:errorcluster, "AvailElmntsForRead"=w563:i32)
        n227 = Greater Than 0?(x=w563) -> (x > 0?=w562:bool)
        n228 = case shown="True" w562 {
          tunnel: [w571 w586] -> w570
          tunnel: [w572 w585] -> w569
          tunnel: w568 -> [_ w578]
          tunnel: w565 -> [w571 w580]
          tunnel: w564 -> [w572 w579]
          frame False {
          }
          frame True {
            n229 = shared-variable-read(w579, w580) -> (w585:refnum<k21>, w586:errorcluster, w576:i32[])  [unwired: 1 in, 1 out]
            n230 = shared-variable "roboRIO-1256-FRC\\Shared Variable.lvlib\\deHeight"() -> (w573:u16)  [unwired: 1 in, 1 out]
            n231 = feedback #10() -> (w574:i32[][])  [unwired: 1 in]
            n232 = Build Array (concatenate)(w574, w576) -> (w577:i32[][])
            n233 = Index Array(array=w577, index (col)=0 ("disabled index (col)")) -> (element=w583:i32[])  [unwired: 1 in]
            n234 = Array Size(array=w583) -> (size(s)=w582:i32)
            n235 = Equal?(x=w582, y=w573) -> (x = y?=w581:bool)
            n236 = case shown="True" w581 {
              tunnel: w577 -> [w587 w588]
              tunnel: [w587 w589] -> w575
              tunnel: w573 -> [_ w593]
              tunnel: w578 -> [_ w590]
              frame False {
              }
              frame True {
                n237 = Delete From Array(array=w588, length=w593, index (row)=0) -> (array with subset deleted=w589:i32[][])  [unwired: 1 in, 1 out]
                n238 = call "IMAQ ArrayToImage"("Image Pixels (U8)"=w588, "Image"=w590) -> ("Image Out"=→"Gaussian2-1":T1)  [unwired: 8 in, 1 out]
                "Array 5" <- w588
              }
            }
            n239 = feedback-in #10(w575) -> ()
          }
        }
      }
      event "停止应用程序 3": Value Change {
        n240 = event-data() -> ()  [unwired: 1 in, 6 out]
        n241 = Not(x="停止应用程序 6") -> (.not. x?=w598:bool)
        n242 = shared-variable "roboRIO-1256-FRC\\Shared Variable.lvlib\\Active"(w598, error in=w597) -> (error out=w596:errorcluster)
      }
    }
  }
  n243 = call "IMAQ Dispose"("Image"=w106) -> ()  [unwired: 5 in, 1 out]
  n244 = Destroy Stream Endpoint(8:w113, 11:w111) -> (0:→"error out 2":errorcluster)
  n245 = Destroy Stream Endpoint(8:w67, 11:w68) -> (0:w92:errorcluster)
  n246 = call "IMAQ Dispose"("Image"=w73) -> ()  [unwired: 5 in, 1 out]
  n247 = Destroy Stream Endpoint(8:w74, 11:w75) -> (0:w91:errorcluster)
  n248 = Destroy Stream Endpoint(8:w123, 11:w122) -> (0:w93:errorcluster)
  n249 = call "IMAQ Dispose"("Image"=w69) -> ()  [unwired: 5 in, 1 out]
  n250 = Destroy Stream Endpoint(8:w6, 11:w5) -> ()  [unwired: 1 out]
  n251 = call "IMAQ Dispose"("Image"=w22) -> ()  [unwired: 5 in, 1 out]
  n252 = Destroy Stream Endpoint(8:w24, 11:w23) -> (0:w19:errorcluster)
  n253 = call "IMAQ Dispose"("Image"=w79) -> ()  [unwired: 5 in, 1 out]
  n254 = Destroy Stream Endpoint(8:w81, 11:w80) -> (0:w85:errorcluster)
  n255 = call "IMAQ Dispose"("Image"=w44) -> ()  [unwired: 5 in, 1 out]
  n256 = Destroy Stream Endpoint(8:w46, 11:w45) -> (0:w21:errorcluster)
  n257 = call "IMAQ Dispose"("Image"=w43) -> ()  [unwired: 5 in, 1 out]
  n258 = Destroy Stream Endpoint(8:w41, 11:w42) -> (0:w20:errorcluster)
  n259 = Destroy Stream Endpoint(8:w17, 11:w18) -> ()  [unwired: 1 out]
  n260 = call "IMAQ Dispose"("Image"=w66) -> ()  [unwired: 5 in, 1 out]
  n261 = Destroy Stream Endpoint(8:w64, 11:w65) -> (0:w55:errorcluster)
  n262 = call "IMAQ Dispose"("Image"=w119) -> ()  [unwired: 5 in, 1 out]
  n263 = Merge Errors(w93, w92, w91, w85, w55, w21, w20, w19) -> (→"error out":errorcluster)
